vi "Generate Simulated Data.vi"(6 "Acquisition":refnum<queue>, 7 "Bits":bool[][](array[boolean]), 8 "error in (no error)":errorcluster, 10 "Longueur d'onde":dbl, 11 "Loop Count":dbl) -> (0 "error out":errorcluster, 2 "Data Out":variant[](array[variant]), 3 "Disconnected":bool=TRUE)   [LabVIEW 2018, in "Acquisition.lvlib"]
doc: "Generates sample waveforms according to the signal type in the HW Config input."
uses:
  Acquisition.lvlib
  support/Message Queue/Message Cluster.ctl
  <vilib>/DAQmx/write.llb/DAQmx Write (Digital 1D Bool NChan 1Samp 1Line).vi
  <vilib>/DAQmx/read.llb/DAQmx Read (Analog 1D Wfm NChan NSamp).vi
  <vilib>/Analysis/baseanly.llb/Mean (DBL).vi
  <vilib>/Analysis/2dsp.llb/2D Convolution (DBL).vi
  <vilib>/DAQmx/create/channels.llb/DAQmx Create Channel (DO-Digital Output).vi
  <vilib>/DAQmx/miscellaneous.llb/DAQmx Fill In Error Info.vi
  <vilib>/DAQmx/create/channels.llb/DAQmx Create Channel (AI-Voltage-Basic).vi
  <vilib>/DAQmx/configure/timing.llb/DAQmx Timing (Sample Clock).vi
  support/Message Queue/Enqueue Message (Single).vi
  GlobalVariable/GlobalPowerByTime.vi
  GlobalVariable/GlobalPosYbyTime.vi
  GlobalVariable/GlobalPosXbyTime.vi
  GlobalVariable/GlobalProfileByTime.vi
  GlobalVariable/Globalt0.vi
  GlobalVariable/GlobalTensionByTime.vi
  GlobalVariable/GlobalTemperatureByTime.vi
  GlobalVariable/GlobalPredictedPower.vi
  GlobalVariable/GlobalSet0.vi
  GlobalVariable/GlobalTimeStep.vi
  <vilib>/gmath/interp.llb/Create Mesh Grid (2D) (x,y arrays).vi
  support/Message Queue/Message Queue.lvlib
  <vilib>/gmath/NI_Gmath.lvlib
  <vilib>/Analysis/NI_AALPro.lvlib
  <resource>/objmgr/daqmx.rc
  <vilib>/Analysis/NI_AALBase.lvlib
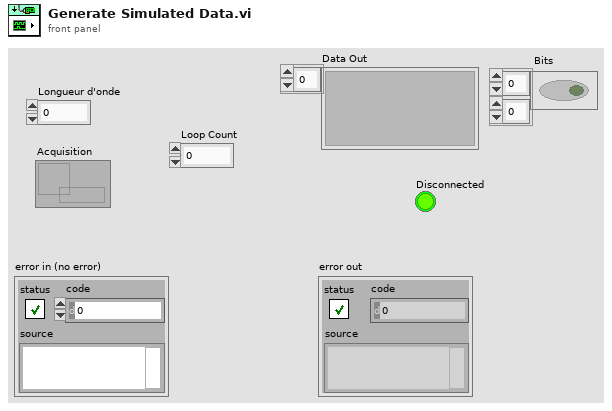
[diagram p1: front panel]
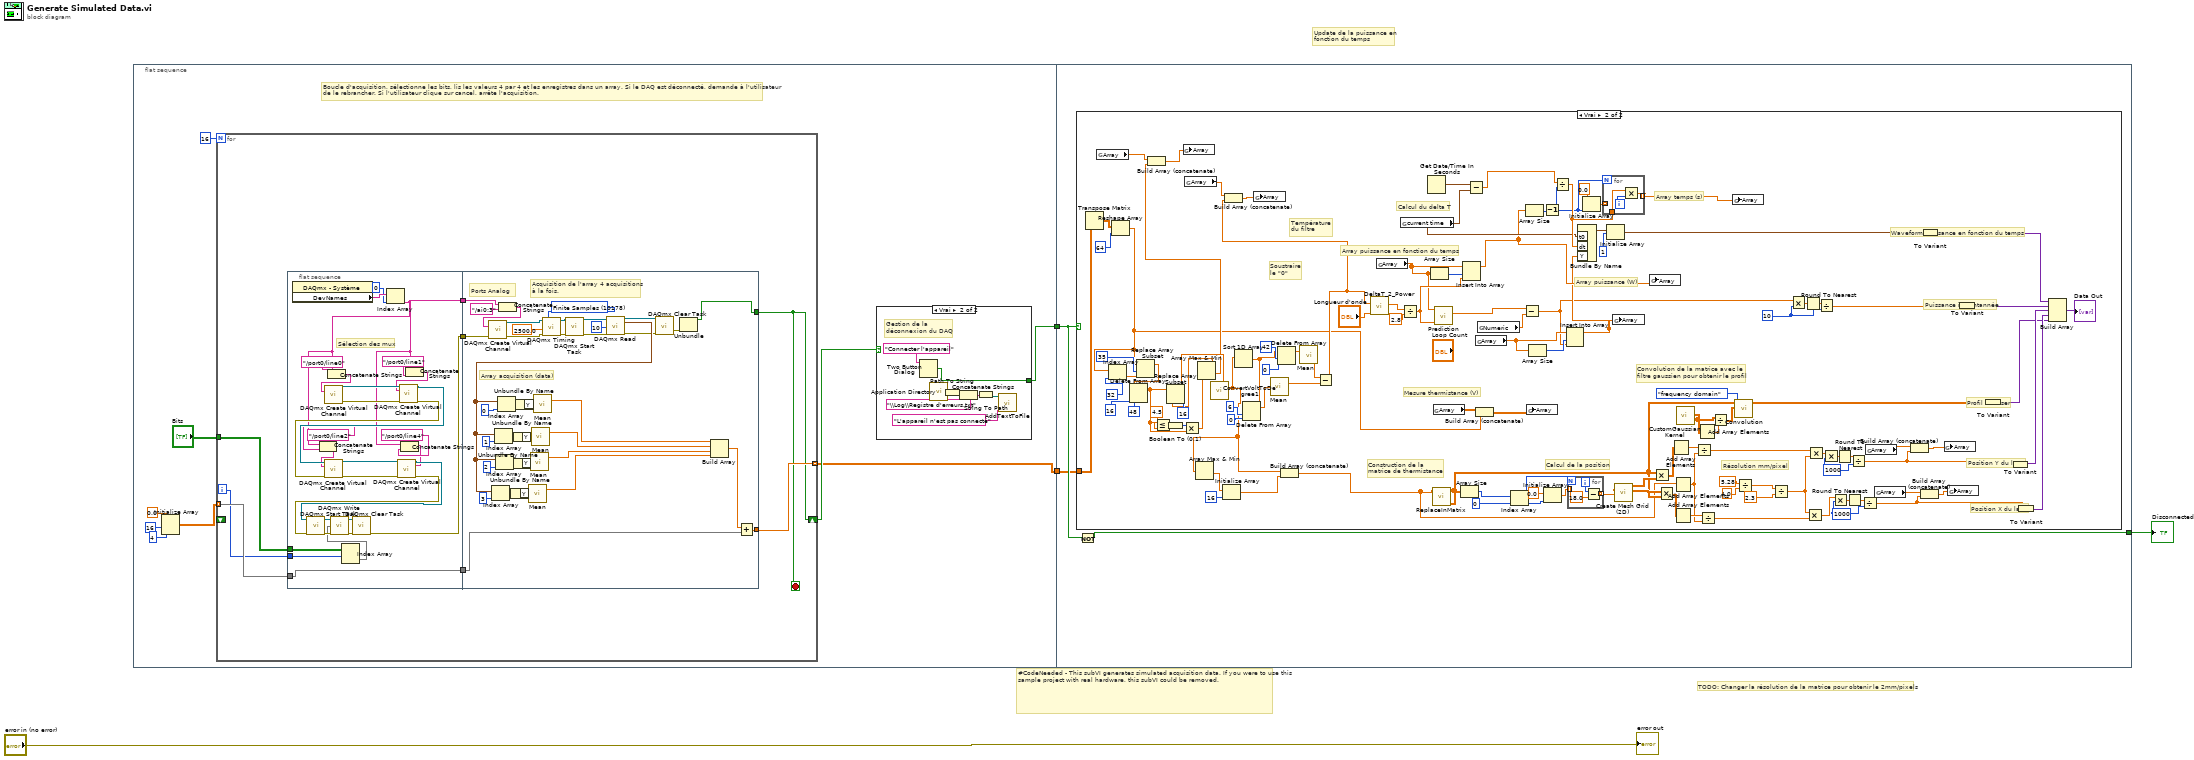
[diagram p0: block diagram]
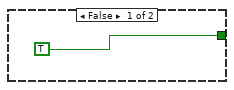
[diagram p2: hidden frame]
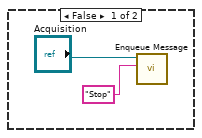
[diagram p3: hidden frame]
diagram:
  # "TODO: Changer la résolution de la matrice pour obtenir le 2mm/pixels"
  # "Update de la puissance en\nfonction du temps"
  # "#CodeNeeded - This subVI generates simulated acquisition data. If you were to use this sample project with real hardware, this subVI could be removed."
  n1 = flat-sequence {
    tunnel: [w9] -> w3
    tunnel: [w7] -> w1
    tunnel: w3 -> [w98]
    tunnel: [w97] -> w2
    tunnel: w1 -> [w96]
    frame #0 {
      # "Boucle d'acquisition, sélectionne les bits, lis les valeurs 4 par 4 et les enregistres dans un array. Si le DAQ est déconnecté, demande à l'utilisateur \nde le rebrancher. Si l'utilisateur clique sur cancel, arrête l'acquisition."
      n2 = Initialize Array(0.0 ("element"), 16 ("dimension size"), 4 ("dimension size")) -> (w10:dbl[][])
      n3 = for {
        N: 16 -> [_]
        tunnel: w10 -> [w30] mode=indexing
        tunnel: [w25] -> w7 mode=indexing
        shift-right: [w24] -> w8
        shift-left: _ -> [_]
        tunnel: "Bits" -> [w23]
        i -> [w26]
        stop <- w24 stop-if-true
        n4 = flat-sequence {
          tunnel: w26 -> [w44]
          tunnel: [w55] -> w29
          tunnel: w23 -> [w43]
          tunnel: [w31] -> w28
          tunnel: [w32] -> w27
          tunnel: w30 -> [w31]
          tunnel: w29 -> [w87]
          tunnel: w28 -> [w67]
          tunnel: [w69] -> w25
          tunnel: w27 -> [w64]
          tunnel: [w59] -> w24
          frame #0 {
            # "Sélection des mux"
            n5 = property class="DAQmx - Système"() -> ("DevNames"=w42:tag[])  [unwired: 2 in, 2 out]
            n6 = Index Array(array=w43, index (row)=w44) -> (element=w56:bool[])  [unwired: 1 in]
            n7 = Index Array(array=w42, index=0) -> (element=w32:tag)
            n8 = Concatenate Strings(w32, "/port0/line2" ("string")) -> (w35:string)
            n9 = Concatenate Strings(w32, "/port0/line0" ("string")) -> (w40:string)
            n10 = call-poly <vilib>:"DAQmx Create Virtual Channel.vi"("lines"=w40) -> ("task out"=w51:refnum<k21>, "error out"=w52:errorcluster)  [unwired: 13 in]
            n11 = Concatenate Strings(w32, "/port0/line4" ("string")) -> (w33:string)
            n12 = Concatenate Strings(w32, "/port0/line1" ("string")) -> (w37:string)
            n13 = call-poly <vilib>:"DAQmx Create Virtual Channel.vi"("task in"=w51, "lines"=w37, "error in"=w52) -> ("task out"=w50:refnum<k21>, "error out"=w49:errorcluster)  [unwired: 11 in]
            n14 = call-poly <vilib>:"DAQmx Create Virtual Channel.vi"("task in"=w50, "lines"=w35, "error in"=w49) -> ("task out"=w47:refnum<k21>, "error out"=w48:errorcluster)  [unwired: 11 in]
            n15 = call-poly <vilib>:"DAQmx Create Virtual Channel.vi"("task in"=w47, "lines"=w33, "error in"=w48) -> ("task out"=w46:refnum<k21>, "error out"=w45:errorcluster)  [unwired: 11 in]
            n16 = call <vilib>:"DAQmx Start Task.vi"("task/channels in"=w46, "error in"=w45) -> ("task out"=w57:refnum<k21>, "error out"=w58:errorcluster)  [unwired: 12 in]
            n17 = call-poly <vilib>:"DAQmx Write.vi"("task/channels in"=w57, "data"=w56, "error in"=w58) -> ("task out"=w54:refnum<k21>, "error out"=w53:errorcluster)  [unwired: 10 in, 1 out]
            n18 = call <vilib>:"DAQmx Clear Task.vi"("task in"=w54, "error in"=w53) -> ("error out"=w55:errorcluster)  [unwired: 13 in]
          }
          frame #1 {
            w89 = 10178 items=["Finite Samples"=10178, "Continuous Samples"=10123, "Hardware Timed Single Point"=12522] ("sample mode")
            # "Ports Analog"
            # "Array acquisition (data)"
            # "Acquisition de l'array 4 acquisitions\nà la fois."
            n19 = Concatenate Strings(w64, "/ai0:3" ("string")) -> (w65:string)
            n20 = call-poly <vilib>:"DAQmx Create Virtual Channel.vi"("physical channels"=w65, "error in"=w87) -> ("task out"=w94:refnum<k21>, "error out"=w93:errorcluster)  [unwired: 12 in]
            n21 = call-poly <vilib>:"DAQmx Timing.vi"("task/channels in"=w94, "sample mode"=w89, "rate"=2500.0, "error in"=w93) -> ("task out"=w90:refnum<k21>, "error out"=w91:errorcluster)  [unwired: 10 in]
            n22 = call <vilib>:"DAQmx Start Task.vi"("task/channels in"=w90, "error in"=w91) -> ("task out"=w92:refnum<k21>, "error out"=w95:errorcluster)  [unwired: 12 in]
            n23 = call-poly <vilib>:"DAQmx Read.vi"("task/channels in"=w92, "number of samples per channel"=10, "error in"=w95) -> ("task out"=w71:refnum<k21>, "data"=w80:waveform(dbl)[], "error out"=w70:errorcluster)  [unwired: 10 in]
            n24 = Index Array(array=w80, index=3) -> (element=w76:waveform(dbl))
            n25 = Index Array(array=w80, index=1) -> (element=w78:waveform(dbl))
            n26 = Index Array(array=w80, index=2) -> (element=w77:waveform(dbl))
            n27 = Index Array(array=w80, index=0) -> (element=w79:waveform(dbl))
            n28 = Unbundle By Name(w76) -> ("Y"=w72:dbl[])
            n29 = Unbundle By Name(w78) -> ("Y"=w74:dbl[])
            n30 = Unbundle By Name(w77) -> ("Y"=w73:dbl[])
            n31 = Unbundle By Name(w79) -> ("Y"=w75:dbl[])
            n32 = call-poly <vilib>:"Mean.vi"("X"=w72) -> ("mean"=w60:dbl)  [unwired: 1 out]
            n33 = call-poly <vilib>:"Mean.vi"("X"=w73) -> ("mean"=w61:dbl)  [unwired: 1 out]
            n34 = call-poly <vilib>:"Mean.vi"("X"=w74) -> ("mean"=w62:dbl)  [unwired: 1 out]
            n35 = call-poly <vilib>:"Mean.vi"("X"=w75) -> ("mean"=w63:dbl)  [unwired: 1 out]
            n36 = call <vilib>:"DAQmx Clear Task.vi"("task in"=w71, "error in"=w70) -> ("error out"=w85:errorcluster)  [unwired: 13 in]
            n37 = Unbundle(w85) -> ("status"=w59:bool)  [unwired: 2 out]
            n38 = Build Array(w63, w62, w61, w60) -> (w68:dbl[])
            n39 = Add(x=w68, y=w67) -> (x+y=w69:dbl[])
          }
        }
      }
      n40 = case shown="Vrai" w8 {
        tunnel: [TRUE w22] -> w9
        frame False {
        }
        frame True {
          # "Gestion de la \ndéconnexion du DAQ"
          n41 = Two Button Dialog(message="Connecter l'appareil") -> (T button?=w22:bool)  [unwired: 2 in]
          n42 = call <vilib>:"Application Directory.vi"() -> ("Application Directory"=w19:path)
          n43 = Path To String(path=w19) -> (string=w20:string)
          n44 = Concatenate Strings(w20, "\\Log\\Registre d'erreurs.txt") -> (w21:string)
          n45 = String To Path(string=w21) -> (path=w15:path)
          n46 = call "AddTextToFile.vi"("Ajouter du texte"="L'appareil n'est pas connecté", "Fichier"=w15) -> ()  [unwired: 10 in]
        }
      }
    }
    frame #1 {
      n47 = case shown="Vrai" w98 {
        tunnel: w96 -> [_ w147]
        frame False {
          n48 = call-poly "Enqueue Message.vi"("Message"="Stop", "Message Queue"="Acquisition") -> ()  [unwired: 8 in, 2 out]
        }
        frame True {
          w177 = 1000
          w181 = 1000
          w187 = 10
          # "Résolution mm/pixel"
          # "Calcul du delta T"
          # "Mesure thermistance (V)"
          # "Soustraire\nle \"0\""
          # "Température \ndu filtre"
          # "Calcul de la position"
          # "Construction de la \nmatrice de thermistance"
          # "Position X du laser"
          # "Position Y du laser"
          # "Profil du laser"
          # "Puissance instantannée"
          # "Waveform puissance en fonction du temps"
          # "Array puissance (W)"
          # "Array temps (s)"
          # "Convolution de la matrice avec le \nfiltre gaussien pour obtenir le profil"
          # "Array puissance en fonction du temps"
          n49 = Transpose Matrix(1:w147) -> (0:w149:dbl[][])
          n50 = global read "GlobalTensionByTime.vi" "Array"() -> (w158:dbl[])
          n51 = Reshape Array(w149, 64 ("dimension size")) -> (w113:dbl[])
          n52 = Index Array(array=w113, index=32) -> (element=w126:dbl)
          n53 = Replace Array Subset(array=w113, new element=w126, index=35) -> (w137:dbl[])
          n54 = Delete From Array(array=w137, length=16, index=48) -> (array with subset deleted=w136:dbl[])  [unwired: 1 out]
          n55 = Less Or Equal?(x=w136, y=4.5) -> (x <= y?=w141:bool[])
          n56 = Boolean To (0,1)(Boolean=w141) -> (0, 1=w140:i16[])
          n57 = Multiply(x=w140, y=w136) -> (x*y=w139:dbl[])
          n58 = global read "GlobalTemperatureByTime.vi" "Array"() -> (w155:dbl[])
          n59 = Array Max & Min(array=w139) -> (max value=w135:dbl, min value=w125:dbl)  [unwired: 2 out]
          n60 = Build Array (concatenate)(w158, w125) -> (w157:dbl[])
          n61 = Replace Array Subset(array=w136, new element=w135, index=16) -> (w127:dbl[])
          n62 = global write "GlobalTensionByTime.vi" "Array"(w157) -> ()
          n63 = call "ConvertVoltToDegree1.vi"("Tension"=w127) -> ("Température"=w108:dbl[])  [unwired: 10 in]
          n64 = Array Max & Min(array=w108) -> (min value=w123:dbl)  [unwired: 3 out]
          n65 = Initialize Array(w123, 16 ("dimension size")) -> (w122:dbl[])
          n66 = Sort 1D Array(array=w108) -> (sorted array=w107:dbl[])
          n67 = Delete From Array(array=w107, length=6, index=0) -> (array with subset deleted=w129:dbl[])  [unwired: 1 out]
          n68 = call-poly <vilib>:"Mean.vi"("X"=w129) -> ("mean"=w104:dbl)  [unwired: 1 out]
          n69 = Delete From Array(array=w107, length=42, index=0) -> (array with subset deleted=w132:dbl[])  [unwired: 1 out]
          n70 = Build Array (concatenate)(w108, w122) -> (w121:dbl[])
          n71 = call-poly <vilib>:"Mean.vi"("X"=w132) -> ("mean"=w128:dbl)  [unwired: 1 out]
          n72 = Subtract(x=w128, y=w104) -> (x-y=w119:dbl)
          n73 = Build Array (concatenate)(w155, w119) -> (w156:dbl[])
          n74 = global write "GlobalTemperatureByTime.vi" "Array"(w156) -> ()
          n75 = call "DeltaT_2_Power.vi"("Longueur d'onde"="Longueur d'onde", "Delta T"=w119) -> ("Power"=w118:dbl)  [unwired: 9 in]
          n76 = global read "GlobalPowerByTime.vi" "Array"() -> (w109:dbl[])
          n77 = global read "Globalt0.vi" "current time"() -> (w160:timestamp)
          n78 = Divide(x=w118, y=2.8) -> (x/y=w116:dbl)
          n79 = Get Date/Time In Seconds() -> (seconds since 1Jan1904=w161:timestamp)
          n80 = Array Size(array=w109) -> (size(s)=w215:i32)
          n81 = call "ReplaceInMatrix.vi"("Input Array"=w121) -> ("Output Array"=w151:dbl[][])  [unwired: 10 in]
          n82 = global read "GlobalProfileByTime.vi" "Array"() -> (w164:dbl[][])
          n83 = call "Prediction.vi"("Puissance Live"=w116, "Puissance prédédente"=w109) -> ("Puissance Prédite"=w102:dbl)  [unwired: 9 in]
          n84 = Array Size(array=w151) -> (size(s)=w208:i32[])
          n85 = Insert Into Array(array=w109, index=w215, new element=w116) -> (w106:dbl[])
          n86 = Subtract(x=w161, y=w160) -> (x-y=w159:dbl)
          n87 = global read "GlobalPredictedPower.vi" "Array"() -> (w114:dbl[])
          n88 = Build Array (concatenate)(w164, w113) -> (w165:dbl[][])
          n89 = global read "GlobalSet0.vi" "Numeric"() -> (w105:dbl)
          n90 = Index Array(array=w208, index=0) -> (element=w203:i32)
          n91 = Subtract(x=w102, y=w105) -> (x-y=w101:dbl)
          n92 = Array Size(array=w106) -> (size(s)=w163:i32)
          n93 = global write "GlobalProfileByTime.vi" "Array"(w165) -> ()
          n94 = Array Size(array=w114) -> (size(s)=w115:i32)
          n95 = Decrement(x=w163) -> (x-1=w162:i32)
          n96 = Initialize Array(0.0 ("element"), w203) -> (w205:dbl[])
          n97 = Divide(x=w159, y=w162) -> (x/y=w211:dbl)
          n98 = Insert Into Array(array=w114, index=w115, new element=w101) -> (w103:dbl[])
          n99 = for {
            N: w203 -> [_]
            tunnel: w205 -> [_] mode=indexing
            tunnel: [w216] -> w200 mode=indexing
            i -> [w217]
            n100 = Subtract(x=w217, y=18.0) -> (x-y=w216:dbl)
          }
          n101 = Bundle By Name("t0"=w160, "dt"=w211, "Y"=w103) -> (w213:waveform(dbl))  [unwired: 1 in]
          n102 = Initialize Array(0.0 ("element"), w162) -> (w209:dbl[])
          n103 = for {
            N: w162 -> [_]
            tunnel: w211 -> [w220]
            tunnel: w209 -> [_] mode=indexing
            tunnel: [w219] -> w172 mode=indexing
            i -> [w221]
            n104 = Multiply(x=w220, y=w221) -> (x*y=w219:dbl)
          }
          n105 = Initialize Array(w213, 1) -> (w191:waveform(dbl)[])
          n106 = global write "GlobalPredictedPower.vi" "Array"(w103) -> ()
          n107 = call-poly <vilib>:"Create Mesh Grid (2D).vi"("y domain"=w200, "x domain"=w200) -> ("Y"=w199:dbl[][], "X"=w204:dbl[][])  [unwired: 7 in, 1 out]
          n108 = global write "GlobalPowerByTime.vi" "Array"(w106) -> ()
          n109 = Multiply(x=w151, y=w204) -> (x*y=w202:dbl[][])
          n110 = Multiply(x=w199, y=w151) -> (x*y=w198:dbl[][])
          n111 = Add Array Elements(numeric array=w202) -> (sum=w201:dbl)
          n112 = Add Array Elements(numeric array=w121) -> (sum=w196:dbl)
          n113 = Add Array Elements(numeric array=w198) -> (sum=w197:dbl)
          n114 = call "CustomGaussianKernel.vi"() -> ("array"=w111:dbl[][])  [unwired: 11 in]
          n115 = Divide(x=w201, y=w196) -> (x/y=w194:dbl)
          n116 = Add Array Elements(numeric array=w111) -> (sum=w112:dbl)
          n117 = Divide(x=w197, y=w196) -> (x/y=w195:dbl)
          n118 = Divide(x=w111, y=w112) -> (x/y=w110:dbl[][])
          n119 = global write "GlobalTimeStep.vi" "Array"(w172) -> ()
          n120 = call-poly <vilib>:"Convolution.vi"("algorithm"=enum32{"direct", "frequency domain"}."frequency domain", "Y"=w110, "X"=w151) -> ("X * Y"=w152:dbl[][])  [unwired: 7 in, 1 out]
          n121 = Divide(x=5.28, y=4.0) -> (x/y=w154:dbl)
          n122 = Divide(x=w154, y=2.3) -> (x/y=w153:dbl)
          n123 = Multiply(x=w101, y=w187) -> (x*y=w188:dbl)
          n124 = Round To Nearest(number=w188) -> (nearest integer value=w186:dbl)
          n125 = Multiply(x=w153, y=w195) -> (x*y=w174:dbl)
          n126 = Multiply(x=w194, y=w153) -> (x*y=w178:dbl)
          n127 = Divide(x=w186, y=w187) -> (x/y=w182:dbl)
          n128 = Multiply(x=w178, y=w181) -> (x*y=w180:dbl)
          n129 = Multiply(x=w174, y=w177) -> (x*y=w176:dbl)
          n130 = Round To Nearest(number=w180) -> (nearest integer value=w179:dbl)
          n131 = Round To Nearest(number=w176) -> (nearest integer value=w175:dbl)
          n132 = Divide(x=w179, y=w181) -> (x/y=w166:dbl)
          n133 = Divide(x=w175, y=w177) -> (x/y=w170:dbl)
          n134 = global read "GlobalPosXbyTime.vi" "Array"() -> (w167:dbl[])
          n135 = global read "GlobalPosYbyTime.vi" "Array"() -> (w171:dbl[])
          n136 = Build Array (concatenate)(w167, w166) -> (w168:dbl[])
          n137 = Build Array (concatenate)(w171, w170) -> (w169:dbl[])
          n138 = To Variant(anything=w191) -> (Variant=w190:variant)
          n139 = global write "GlobalPosXbyTime.vi" "Array"(w168) -> ()
          n140 = global write "GlobalPosYbyTime.vi" "Array"(w169) -> ()
          n141 = To Variant(anything=w182) -> (Variant=w183:variant)
          n142 = To Variant(anything=w152) -> (Variant=w173:variant)
          n143 = To Variant(anything=w166) -> (Variant=w184:variant)
          n144 = To Variant(anything=w170) -> (Variant=w185:variant)
          n145 = Build Array(w190, w183, w184, w185, w173) -> (→"Data Out":variant[])
        }
      }
      n146 = Not(x=w98) -> (.not. x?=w97:bool)
    }
  }
  "error out" <- "error in (no error)"
  "Disconnected" <- w2
